vi "last_array_element.vi"(1 "Array":cluster{"X":i32, "Y":i32}[](array[cluster])) -> (0 "Last Element":cluster{"X":i32, "Y":i32})   [LabVIEW 2017]
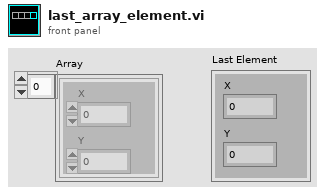
[diagram p1: front panel]
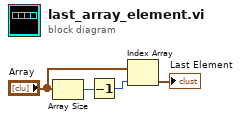
[diagram p0: block diagram]
diagram:
  n1 = Array Size(array="Array") -> (size(s)=w4:i32)
  n2 = Decrement(x=w4) -> (x-1=w3:i32)
  n3 = Index Array(array="Array", index=w3) -> (element=→"Last Element":cluster{"X":i32, "Y":i32})
